vi "AG Get Path.vi"(5 "ignore case? (T)":bool=TRUE, 7 "Partial File Name":string, 9 "error in (no error)":errorcluster, 10 "Resources":path[](array[path])) -> (1 "error out":errorcluster, 2 "Path":path, 4 "Found?":bool, 6 "Resources Directory":path)   [LabVIEW 2012]
doc: "Find a specific item in the resource directory from a page in a LabVIEW Activity Guide."
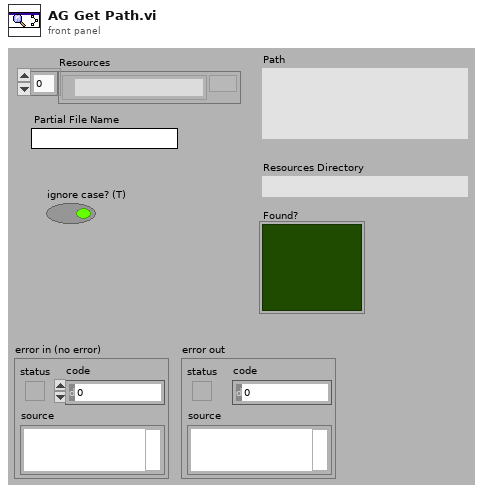
[diagram p1: front panel]
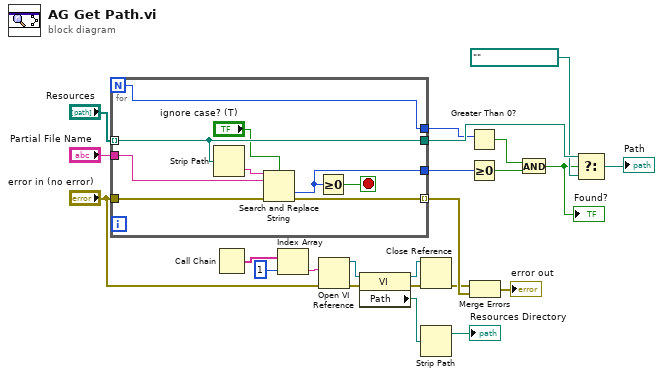
[diagram p0: block diagram]
diagram:
  n1 = for {
    N -> [w24]
    tunnel: "Resources" -> [w31] mode=indexing
    tunnel: "Partial File Name" -> [w29]
    tunnel: [w28] -> w21
    tunnel: [w31] -> w19
    tunnel: "error in (no error)" -> [w26]
    tunnel: [w25] -> w9 mode=indexing
    tunnel: [w24] -> w3
    stop <- w32 stop-if-true
    n2 = Strip Path(path=w31) -> (name=w30:string)  [unwired: 1 out]
    n3 = Search and Replace String(case sensitive?="ignore case? (T)", input string=w30, search string=w29, error in=w26) -> (offset past replacement=w28:i32, error out=w25:errorcluster)  [unwired: 4 in, 2 out]
    n4 = Greater Or Equal To 0?(x=w28) -> (x >= 0?=w32:bool)
  }
  n5 = Call Chain() -> (call chain=w16:string[])
  n6 = Index Array(array=w16, index=1) -> (element=w14:string)
  n7 = Open VI Reference(vi path=w14, error in (no error)="error in (no error)") -> (vi reference=w13:refnum<vi>, error out=w11:errorcluster)  [unwired: 4 in]
  n8 = property class="VI"(reference=w13, error in=w11) -> (reference out=w8:refnum<vi>, error out=w6:errorcluster, "Path"=w12:path)
  n9 = Close Reference(reference=w8, error in (no error)=w6) -> (error out=w5:errorcluster)
  n10 = Strip Path(path=w12) -> (stripped path=→"Resources Directory":path)  [unwired: 1 out]
  n11 = Greater Than 0?(x=w3) -> (x > 0?=w2:bool)
  n12 = Greater Or Equal To 0?(x=w21) -> (x >= 0?=w4:bool)
  n13 = Merge Errors(w5, w9) -> (→"error out":errorcluster)
  n14 = And(x=w2, y=w4) -> (x .and. y?=w1:bool)
  "Found?" <- w1
  n15 = Select(t=w19, s=w1, f=path "" ("t")) -> (s? t:f=→"Path":path)
